vi "FTW-Request-Reply.vi"(0 "FTW Incoming Request":refnum<class "FTW-Request.lvclass">, 5 "Send Timeout":i32 format="%dmsec", 11 "error in":errorcluster) -> (6 "Timed out?":bool, 15 "error out":errorcluster)   [LabVIEW 2013, in "FTW-Request.lvclass"]
doc: "Sends a response message back to the requesting client. This message is attempts to send unconditionally of incoming error. Take caution to wire a sanitized error into this function, because it will be repeated back onto the client. Said another way, an error generated while processing the request will be not only thrown on the request handler, but also on the client as well."
uses:
  FTW-Request.lvclass
  FTW-Request.lvclass/FTW-Request.ctl
  json/FTW-JSON.lvclass
  message/FTW-Message.lvclass
panel:
  # "Inputs"
  # "Outputs"
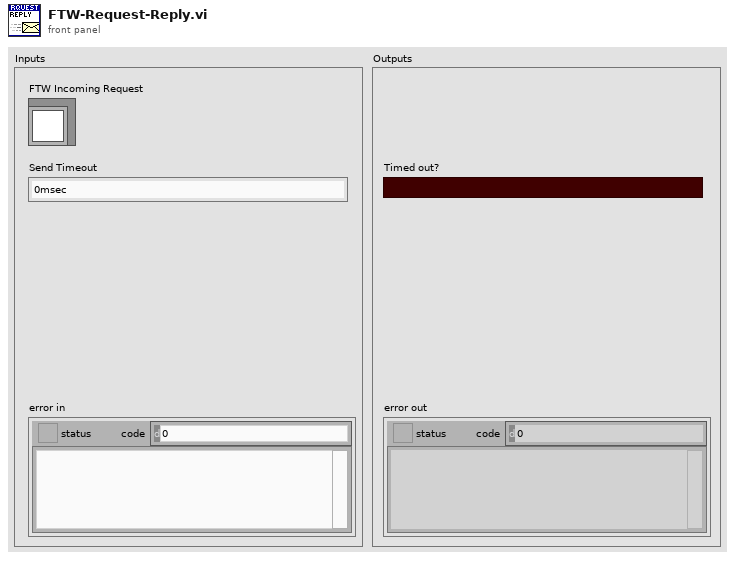
[diagram p1: front panel]
types:
  T1 = typedef "FTW-ERR-ExceptionType.ctl" = enum16{"OK", "Error", "Warning"}
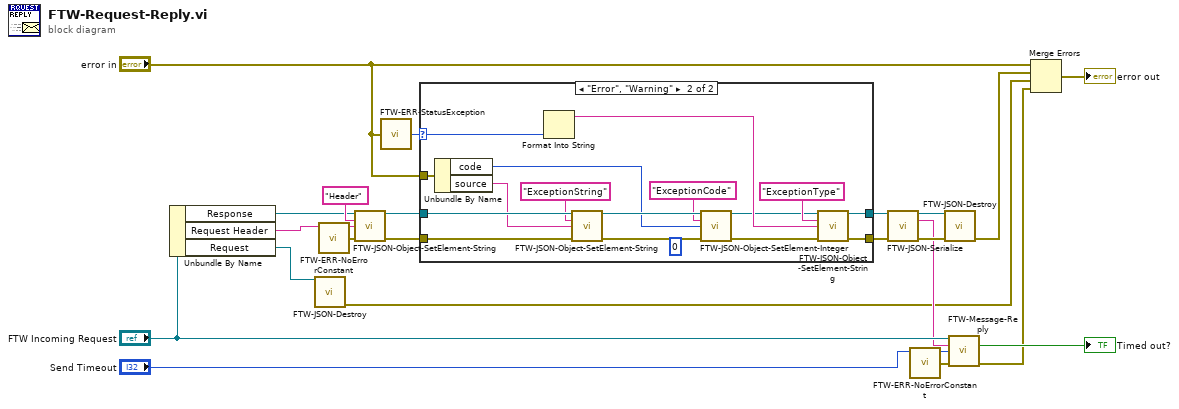
[diagram p0: block diagram]
diagram:
  n1 = Unbundle By Name("FTW Incoming Request") -> ("Response"=w7:refnum<class "FTW-JSON.lvclass">, "Request Header"=w3:string, "Request"=w12:refnum<class "FTW-JSON.lvclass">)
  n2 = call "FTW-JSON-Destroy.vi"("JSON Object"=w12) -> ("error out"=w11:errorcluster)  [unwired: 14 in]
  n3 = call "FTW-ERR-NoErrorConstant.vi"() -> ("no error"=w5:errorcluster)
  n4 = call "FTW-JSON-Object-SetElement-String.vi"("JSON Object"=w7, "Key"="Header", "Value"=w3, "error in"=w5) -> ("JSON Object out"=w6:refnum<class "FTW-JSON.lvclass">, "error out"=w4:errorcluster)  [unwired: 10 in]
  n5 = call "FTW-ERR-StatusException.vi"("error to check"="error in") -> ("Exception"=w2:T1)
  n6 = case shown="\"Error\", \"Warning\"" w2 {
    selector: w2 -> [_ w37]
    tunnel: w6 -> [w24 w40]
    tunnel: [w24 w36] -> w19
    tunnel: [w23 w35] -> w18
    tunnel: w4 -> [w23 w38]
    tunnel: "error in" -> [_ w30]
    frame "OK" {
    }
    frame "Error", "Warning" {
      (unwired) 0 ("code")
      n7 = Unbundle By Name(w30) -> ("code"=w29:i32, "source"=w27:string)
      n8 = Format Into String(w37) -> (resulting string=w33:string)  [unwired: 3 in, 1 out]
      n9 = call "FTW-JSON-Object-SetElement-String.vi"("JSON Object"=w40, "Key"="ExceptionString", "Value"=w27, "error in"=w38) -> ("JSON Object out"=w32:refnum<class "FTW-JSON.lvclass">, "error out"=w26:errorcluster)  [unwired: 10 in]
      n10 = call "FTW-JSON-Object-SetElement-Integer.vi"("JSON Object"=w32, "Key"="ExceptionCode", "Value"=w29, "error in"=w26) -> ("JSON Object out"=w31:refnum<class "FTW-JSON.lvclass">, "error out"=w25:errorcluster)  [unwired: 10 in]
      n11 = call "FTW-JSON-Object-SetElement-String.vi"("JSON Object"=w31, "Key"="ExceptionType", "Value"=w33, "error in"=w25) -> ("JSON Object out"=w36:refnum<class "FTW-JSON.lvclass">, "error out"=w35:errorcluster)  [unwired: 10 in]
    }
  }
  n12 = call "FTW-JSON-Serialize.vi"("JSON Object"=w19, "error in"=w18) -> ("JSON Object out"=w22:refnum<class "FTW-JSON.lvclass">, "JSON String (UTF-8)"=w16:string, "error out"=w21:errorcluster)  [unwired: 11 in]
  n13 = call "FTW-ERR-NoErrorConstant.vi"() -> ("no error"=w13:errorcluster)
  n14 = call "FTW-JSON-Destroy.vi"("JSON Object"=w22, "error in"=w21) -> ("error out"=w15:errorcluster)  [unwired: 13 in]
  n15 = call "FTW-Message-Reply.vi"("FTW Incoming Message"="FTW Incoming Request", "Response"=w16, "Send Timeout"="Send Timeout", "error in"=w13) -> ("Timed out?"=→"Timed out?":bool, "error out"=w10:errorcluster)  [unwired: 10 in]
  n16 = Merge Errors("error in", w15, w11, w10) -> (→"error out":errorcluster)
